vi "Arduino_Answer.vi"() -> ()   [LabVIEW 2018]
panel:
  out "output 1":dbl
  out "return count":u32
  out "error out":errorcluster
  out "read buffer":string
  in  "baud rate (115200)":u32=115200
  in  "VISA resource name":refnum<visa-resource-name>
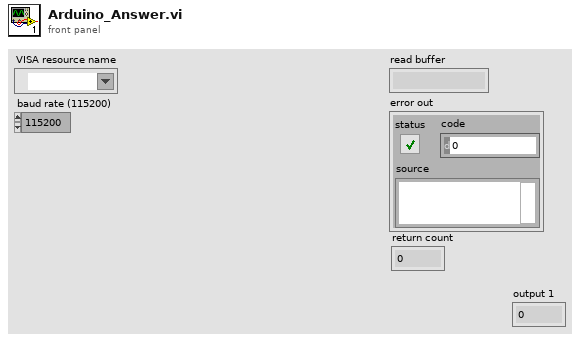
[diagram p1: front panel]
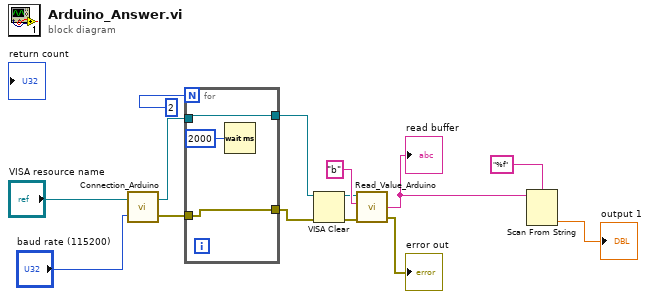
[diagram p0: block diagram]
diagram:
  n1 = call "Connection_Arduino.vi"("Baud rate (115200)"="baud rate (115200)", "VISA resource name"="VISA resource name") -> ("error out"=w2:errorcluster, "VISA resource name out"=w4:refnum<visa-resource-name>)
  n2 = for {
    N: 2 -> [_]
    tunnel: w4 -> [w16]
    tunnel: [w16] -> w3
    tunnel: w2 -> [w15]
    tunnel: [w15] -> w1
    n3 = Wait (ms)(milliseconds to wait=u32 2000) -> ()  [unwired: 1 out]
  }
  n4 = VISA Clear(VISA resource name=w3, error in (no error)=w1) -> (VISA resource name out=w10:refnum<visa-resource-name>, error out=w9:errorcluster)
  n5 = call "Read_Value_Arduino.vi"("error in (no error)"=w9, "write buffer"="b", "VISA resource name"=w10) -> ("error out"=→"error out":errorcluster, "concatenated string"=w7:string)  [unwired: 1 in, 1 out]
  "read buffer" <- w7
  n6 = Scan From String(format string="%f", input string=w7) -> (output 1=→"output 1":dbl)  [unwired: 3 in, 3 out]
